vi "Labview_to_unity_2.vi"   [LabVIEW 2017]
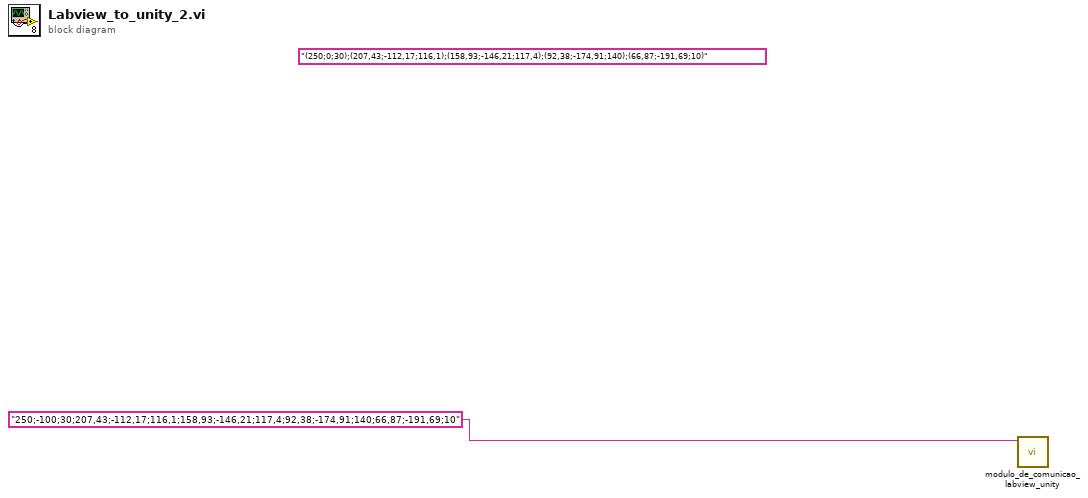
[diagram p0: block diagram]
diagram:
  (unwired) "(250;0;30);(207,43;-112,17;116,1);(158,93;-146,21;117,4);(92,38;-174,91;140);(66,87;-191,69;10)"
  n1 = call "modulo_de_comunicao_labview_unity.vi"("String"="250;-100;30;207,43;-112,17;116,1;158,93;-146,21;117,4;92,38;-174,91;140;66,87;-191,69;10") -> ()  [unwired: 11 in]
